vi "Write Whole SEQ.vi"(4 "Header file data":T1 {"Pixel depth" items=["8 bits", "16 bits", "Float", "Complex", "RGB", "HSL"]; "time of 1st frame, \nsec since 1/1/04" format="%.2f"}, 5 "AOI List":u16[][](array[numeric]), 6 "Acqisition files refnums":refnum<file>[](array[refnum]), 7 "error in":errorcluster, 8 "Number of images":u32, 9 "SEQ file refnum":refnum<file>, 10 "First image number":u32) -> (0 "error out":errorcluster)   [LabVIEW 2016]
doc: "Write Whole SEQ.vi\n\nConverts a series of images to the SEQ format. The number of images is retrieved by array sizing the image array."
uses:
  Header file data.ctl
  Seq file v 1/Offset table.ctl
  Seq file v 1/Offset.ctl
  Seq file v 1/file number.ctl
panel:
  in  "stop":bool
  out "Progress":u32(slide) scale=1.0..61.0
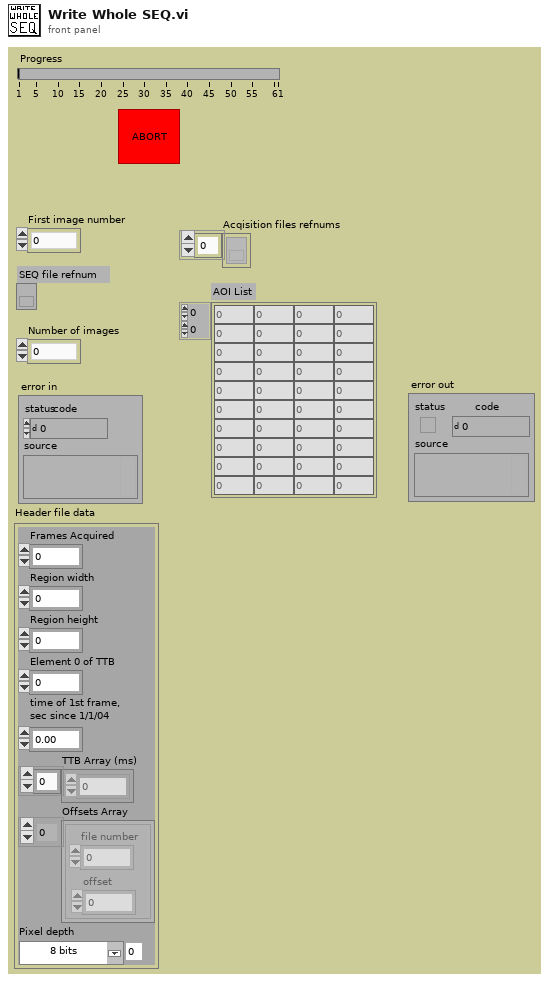
[diagram p1: front panel]
types:
  T1 = typedef "Header file data.ctl" = cluster{"Frames Acquired":u32, "Region width":i32, "Region height":i32, "Element 0 of TTB":u32, "time of 1st frame, \nsec since 1/1/04":dbl, "TTB Array (ms)":u32[], "Offsets Array":T2, "Pixel depth":u32}
  T2 = typedef "Offset table.ctl" = cluster{"offset":T3, "file number":T4}[]
  T3 = typedef "Offset.ctl" = i32
  T4 = typedef "file number.ctl" = u8
  T5 = enum32{"8 bits", "16 bits", "Float", "Complex", "RGB Chunky", "Compressed"}
  T6 = typedef "IMAQ Image.ctl" = refnum<image>
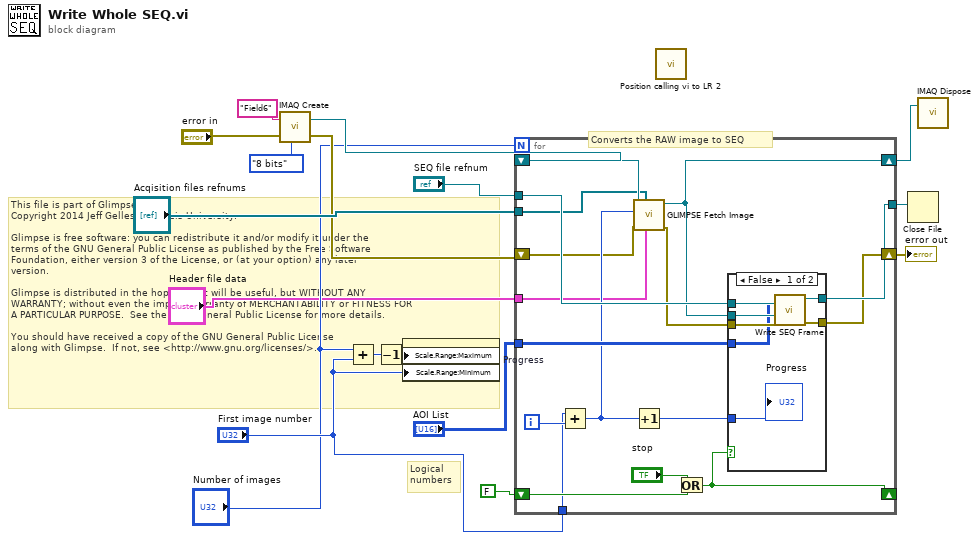
[diagram p0: block diagram]
diagram:
  # "This file is part of Glimpse. \nCopyright 2014 Jeff Gelles, Brandeis University.    \n\nGlimpse is free software: you can redistribute it and/or modify it under the \nterms of the GNU General Public License as published by the Free Software \nFoundation, either version 3 of the License, or (at your option) any later \nversion.\n\nGlimpse is distributed in the hope that it will be useful, but WITHOUT ANY \nWARRANTY; without even the implied warranty of MERCHANTABILITY or FITNESS FOR \nA PARTICULAR PURPOSE.  See the GNU General Public License for more details.\n\nYou should have received a copy of the GNU General Public License\nalong with Glimpse.  If not, see <http://www.gnu.org/licenses/>."
  # "Logical\nnumbers"
  # "Converts the RAW image to SEQ"
  n1 = call "IMAQ Create"("Image Name"="Field6", "Image Type"=T5."8 bits", "error in (no error)"="error in") -> ("New Image"=w11:T6, "error out"=w6:errorcluster)  [unwired: 1 in, 1 out]
  n2 = Add(x="Number of images", y="First image number") -> (x+y=w4:u32)
  n3 = Decrement(x=w4) -> (x-1=w9:u32)
  n4 = property on="Progress" class="Slide (strict)"("Scale.Range:Maximum"=w9, "Scale.Range:Minimum"="First image number") -> ()  [unwired: 2 in, 2 out]
  n5 = for {
    N: "Number of images" -> [_]
    tunnel: "SEQ file refnum" -> [w34]
    tunnel: [w20] -> w16
    tunnel: "AOI List" -> [w33]
    shift-right: [w29] -> _
    shift-left: FALSE -> [w31]
    shift-right: [w24] -> w10
    shift-left: w11 -> [w28]
    tunnel: "First image number" -> [w25]
    tunnel: "Acqisition files refnums" -> [w23]
    shift-right: [w19] -> w5
    shift-left: w6 -> [w22]
    tunnel: "Header file data" -> [w18]
    i -> [w26]
    n6 = Add(x=w25, y=w26) -> (x+y=w27:u32)
    n7 = call "GLIMPSE Fetch Image.vi"("Header file data"=w18, "Acqisition files refnums"=w23, "error in"=w22, "Logical Frame Number\n(starting with zero)"=w27, "Image In"=w28) -> ("error out"=w21:errorcluster, "Image Out"=w24:T6)  [unwired: 2 in, 3 out]
    n8 = Increment(x=w27) -> (x+1=w32:u32)
    n9 = Or(x="stop", y=w31) -> (x .or. y?=w29:bool)
    n10 = case shown="False" w29 {
      tunnel: w34 -> [w41 w43]
      tunnel: w24 -> [w40 _]
      tunnel: w33 -> [w37 _]
      tunnel: w32 -> [w39 _]
      tunnel: w21 -> [w38 w42]
      tunnel: [w36 w43] -> w20
      tunnel: [w35 w42] -> w19
      frame False {
        n11 = call "Write SEQ Frame.vi"("error in (no error)"=w38, "Image In"=w40, "AOI List"=w37, "Seq file refnum"=w41) -> ("error out"=w35:errorcluster, "dup refnum"=w36:refnum<file>)  [unwired: 2 out]
        "Progress" <- w39
      }
      frame True {
      }
    }
  }
  "error out" <- w5
  n12 = call "Position calling vi to LR 2.vi"() -> ()  [unwired: 2 in, 4 out]
  n13 = Close File(refnum=w16) -> ()  [unwired: 1 in, 2 out]
  n14 = call "IMAQ Dispose"("Image"=w10) -> ()  [unwired: 2 in, 4 out]
